vi "Reset Camera on Error.vi"(8 "error in":errorcluster, 10 "Image in":T1, 11 "Session in":T2) -> (0 "error out":errorcluster, 2 "Image out":T1, 3 "Session out":T2)   [LabVIEW 2012, in "Camera SubVIs.lvlib"]
uses:
  Camera SubVIs.lvlib
  <vilib>/userdefined/High Color/IMAQdx.ctl
  <vilib>/vision/Image Controls.llb/IMAQ Image.ctl
  <vilib>/vision/driver/NI_Vision_Acquisition_Software.lvlib
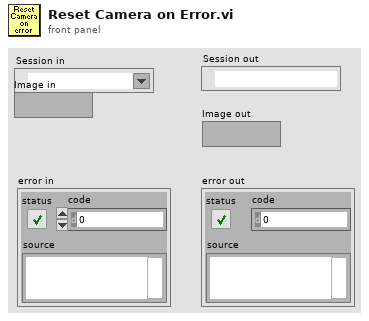
[diagram p1: front panel]
types:
  T1 = typedef "IMAQ Image.ctl" = refnum<image>
  T2 = typedef "IMAQdx.ctl" = refnum<k21>
  T3 = typedef "Image Type" = u32
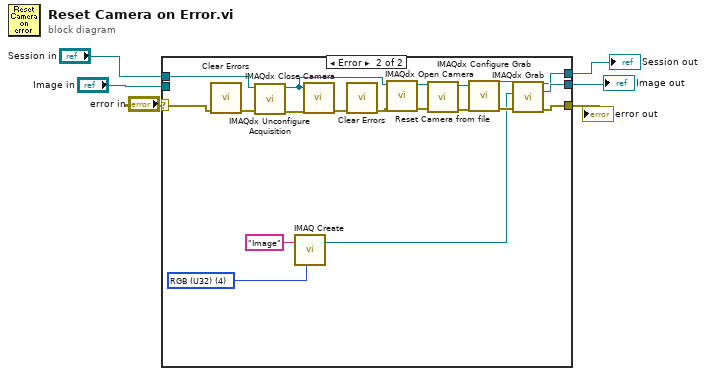
[diagram p0: block diagram]
diagram:
  n1 = case shown="Error" "error in" {
    selector: "error in" -> [w9 w28]
    tunnel: [w9 w26] -> w3
    tunnel: [w8 w24] -> w4
    tunnel: "Image in" -> [w8 _]
    tunnel: "Session in" -> [w7 w18]
    tunnel: [w7 w23] -> w6
    frame No Error {
    }
    frame Error {
      w17 = T3 4 items=["Grayscale (U8)", "Grayscale (I16)", "Grayscale (SGL)", "Complex (CSG)", "RGB (U32)", "HSL (U32)", "RGB (U64)", "Grayscale (U16)"] ("Image Type")
      n2 = call <vilib>:"Clear Errors.vi"("error in (no error)"=w28) -> ("error out"=w20:errorcluster)  [unwired: 6 in]
      n3 = call <vilib>:"IMAQdx Unconfigure Acquisition.vi"("error in"=w20, "Session In"=w18) -> ("error out"=w19:errorcluster, "Session Out"=w14:T2)  [unwired: 8 out]
      n4 = call "IMAQ Create"("Image Name"="Image", "Image Type"=w17) -> ("New Image"=w15:T1)  [unwired: 2 in, 2 out]
      n5 = call <vilib>:"IMAQdx Close Camera.vi"("error in"=w19, "Session In"=w14) -> ("error out"=w22:errorcluster)  [unwired: 9 in]
      n6 = call <vilib>:"Clear Errors.vi"("error in (no error)"=w22) -> ("error out"=w21:errorcluster)  [unwired: 6 in]
      n7 = call <vilib>:"IMAQdx Open Camera.vi"("error in"=w21, "Session In"=w14) -> ("error out"=w12:errorcluster, "Session Out"=w13:T2)  [unwired: 8 in]
      n8 = call "Reset Camera from file.vi"("error in"=w12, "Refnum in"=w13) -> ("error out"=w10:errorcluster, "Refnum out"=w11:T2)  [unwired: 8 in]
      n9 = call <vilib>:"IMAQdx Configure Grab.vi"("error in"=w10, "Session In"=w11) -> ("error out"=w27:errorcluster, "Session Out"=w25:T2)  [unwired: 8 in]
      n10 = call <vilib>:"IMAQdx Grab.vi"("error in"=w27, "Image In"=w15, "Session In"=w25) -> ("error out"=w26:errorcluster, "Image Out"=w24:T1, "Session Out"=w23:T2)  [unwired: 5 in, 1 out]
    }
  }
  "Session out" <- w6
  "Image out" <- w4
  "error out" <- w3
